vi "DotNETCam_GetPicture.vi"(8 "ErrorIn":errorcluster, 10 "CmdData":variant, 11 "DotNETCamIn":refnum<class>) -> (0 "ErrorOut":errorcluster, 2 "ReplyData":variant, 3 "DotNETCamOut":refnum<class>, 4 "Exit":bool)   [LabVIEW 2021, in "DotNETCam.lvclass"]
uses:
  DotNETCam.lvclass
  DotNETCam.lvclass/DotNETCam.ctl
  C:/Localdata/Projects/TriekselSoft/TriekselsoftApplicationFramework/Source/.Externals/Library_YAF/YAFTAF/YAFTAF.lvclass
  C:/Localdata/Projects/TriekselSoft/TriekselsoftApplicationFramework/Source/.Externals/Library_YAF/YActor/YActor.lvclass
  C:/Localdata/Projects/TriekselSoft/TriekselsoftApplicationFramework/Source/.Externals/Interface_UserInterface_IFrontPanel/IFrontPanel/IFrontPanel.lvclass
  C:/Localdata/Projects/TriekselSoft/TriekselsoftApplicationFramework/Source/IInterface/IInterface.lvclass
  C:/Localdata/Projects/TriekselSoft/TriekselsoftApplicationFramework/Source/.Externals/Interface_Object_ICreateDestroy/ICreateDestroy/ICreateDestroy.lvclass
  C:/Localdata/Projects/TriekselSoft/TriekselsoftApplicationFramework/Source/.Externals/Interface_Object_IPersistentData/IPersistentData/IPersistentData.lvclass
  C:/Localdata/Projects/TriekselSoft/TriekselsoftApplicationFramework/Source/.Externals/Interface_TAF_ITAFObject/ITAFObject/ITAFObject.lvclass
  C:/Localdata/Projects/TriekselSoft/TriekselsoftApplicationFramework/Source/YAFTAFObjects/DotNETCam/DotNETCam.lvclass
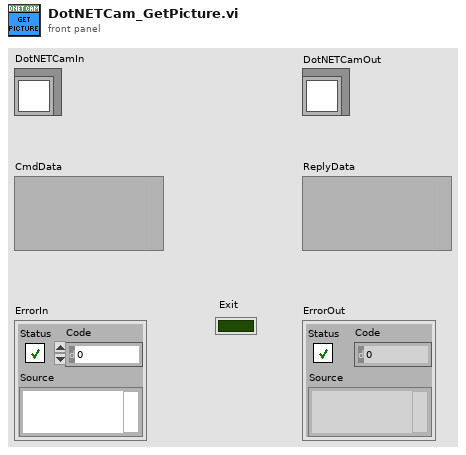
[diagram p1: front panel]
types:
  T1 = typedef "DotNETCam.lvclass/State.ctl" = enum16{"Idle", "Acquiring"}
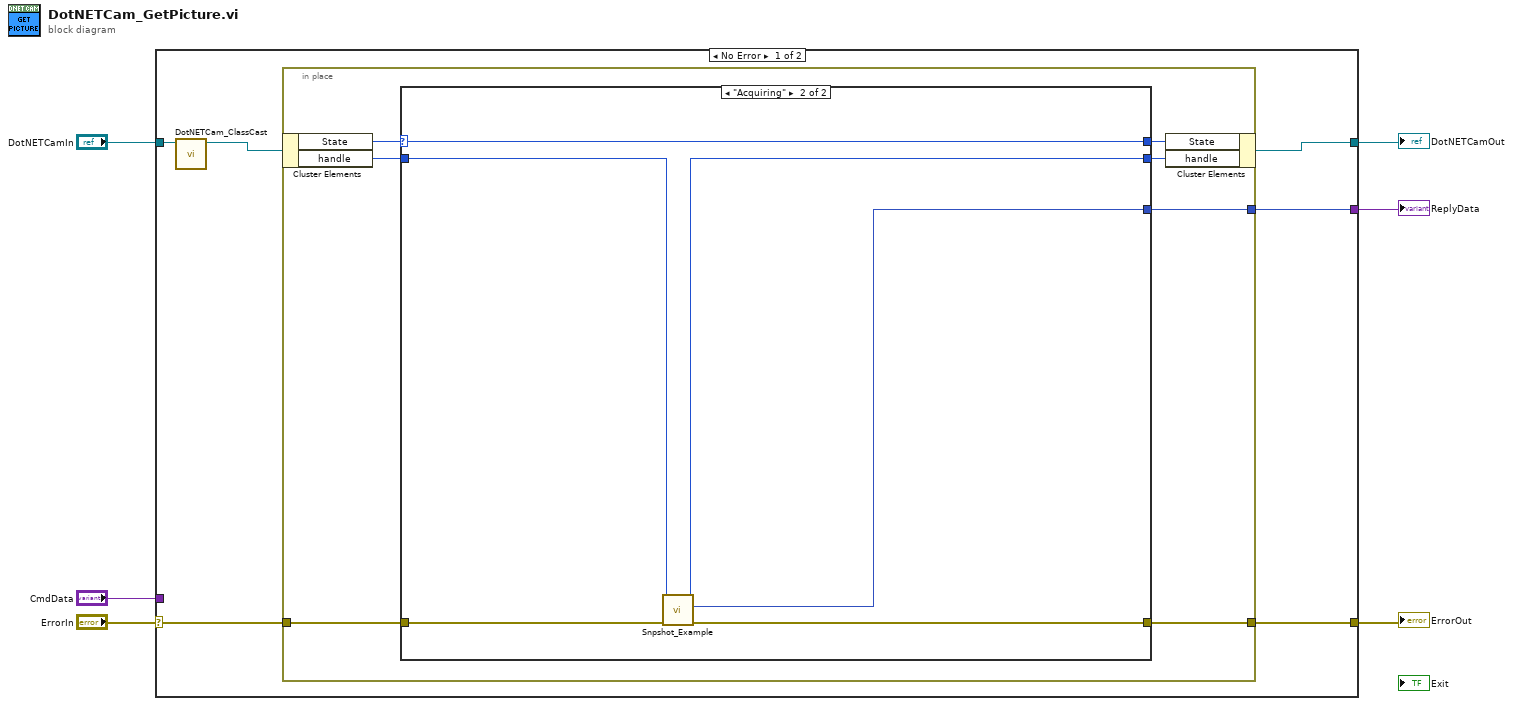
[diagram p0: block diagram]
diagram:
  n1 = case shown="No Error" "ErrorIn" {
    selector: "ErrorIn" -> [w12 w31]
    tunnel: [w11 w31] -> w5
    tunnel: [w7 w30] -> w3
    tunnel: "CmdData" -> [_ w30]
    tunnel: "DotNETCamIn" -> [w10 w29]
    tunnel: [w8 w29] -> w1
    frame No Error {
      n2 = call "DotNETCam_ClassCast.vi"("DotNETCamIn"=w10) -> ("DotNETCamOut"=w9:refnum<class "DotNETCam.lvclass">)  [unwired: 10 in]
      n3 = in-place {
        in-place-border: w12 -> [w19]
        in-place-border: [w18] -> w11
        in-place-border: [w13] -> w7
        n4 = in-place-cluster #1(w9) -> ("State"=w17:T1, "handle"=w14:i32)
        n5 = case shown="\"Acquiring\"" w17 {
          selector: w17 -> [w21 w26]
          tunnel: [w22 w28] -> w18
          tunnel: w19 -> [w22 w27]
          tunnel: [w21 w26] -> w16
          tunnel: [w20 w24] -> w15
          tunnel: w14 -> [w20 w25]
          tunnel: [_ w23] -> w13
          frame "Idle" {
          }
          frame "Acquiring" {
            n6 = call "Snpshot_Example.vi"("ErrorIn"=w27, "Handle"=w25) -> ("ErrorOut"=w28:errorcluster, "Snapshot"=w23:picture, "HandleOut"=w24:i32)  [unwired: 7 in]
          }
        }
        n7 = in-place-cluster #1("State"=w16, "handle"=w15) -> (w8:refnum<class "DotNETCam.lvclass">)
      }
    }
    frame Error {
    }
  }
  "ErrorOut" <- w5
  "DotNETCamOut" <- w1
  "ReplyData" <- w3
